vi "Reuben_Reactor_main_jarryd.vi"() -> ()   [LabVIEW 2018]
uses:
  Labview files/Waldo Labview Files/Control 1.ctl
  Labview files/Waldo Labview Files/Control 2.ctl
  <vilib>/DAQmx/read.llb/DAQmx Read (Analog 1D DBL NChan 1Samp).vi
  <vilib>/DAQmx/write.llb/DAQmx Write (Digital 1D Bool NChan 1Samp 1Line).vi
  <vilib>/DAQmx/write.llb/DAQmx Write (Analog 1D DBL NChan 1Samp).vi
  <vilib>/DAQmx/create/channels.llb/DAQmx Create Channel (AI-Current-Basic).vi
  <vilib>/DAQmx/create/channels.llb/DAQmx Create Channel (AI-Voltage-Basic).vi
  <vilib>/DAQmx/create/channels.llb/DAQmx Create Channel (DO-Digital Output).vi
  <vilib>/DAQmx/create/channels.llb/DAQmx Create Channel (AO-Current-Basic).vi
  <vilib>/DAQmx/miscellaneous.llb/DAQmx Fill In Error Info.vi
  <vilib>/Utility/file.llb/Write To Spreadsheet File (string).vi
panel:
  in  "Offset":dbl
  out "Run time":dbl
  out "x*y":dbl
  in  "Numeric":dbl format="%#_13g"
  in  "Actual RPM":dbl format="%#_13g"
  in  "Nitrogen rpm":dbl format="%#_13g"
  in  "Glucose rpm":dbl format="%#_13g"
  in  "Heating cycle (s)":dbl=5.0 format="%#_13g"
  out "Air Average":dbl
  out "Sample Time (ms)":u32=1000
  out "Time":string
  out "On/Off":bool
  out "O2 % Average":dbl
  out "CO2 % Average":dbl
  out "Python code error out":errorcluster
  in  "Inlet O2 %":dbl format="%#_13g"
  in  "Biomass (g)":dbl format="%#_13g"
  in  "Inlet CO2 %":dbl format="%#_13g"
  in  "Python code":path
  out "Data Outputs":dbl[](array[numeric]) format="%.4f"
  in  "323 Auto":bool
  in  "323 Direction":bool
  out "CO2 Average":dbl
  in  "120U Manual":bool
  in  "120U On/Off":bool
  out "Dosing average":dbl
  out "Pump":bool
  in  "Integrator array size":dbl
  in  "Auto":bool
  in  "Heating fraction":dbl
  in  "Temperature setpoint":dbl
  in  "File path (dialog if empty)":path
  out "Data Inputs":T1 format="%.8f"
  in  "Feed rpm \n(0.4623 ml/min/rpm)":dbl
  in  "Gas Recycle":dbl
  in  "Dosing rpm\n (0.042 ml/min/rpm)":dbl
  in  "Broth Recycle":dbl
  in  "Air (ml/min)":dbl
  in  "CO2 (ml/min)":dbl
  in  "Tab Control":enum32{"10 min", "1 h", "6 h", "24 h", "100 h"}(tab)
  out "Gas analyser O2 % 10 min":dbl(graph)
  out "pH 10 min":dbl(graph)
  out "CO2 Feed 10 min":dbl(graph)
  out "Gas analyser CO2 % 10 min":dbl(graph)
  out "Air Feed 10 min":dbl(graph)
  out "blank":dbl(graph)
  out "Temperature 10 min":dbl(graph)
  out "Dosing 10 min":dbl(graph)
  out "O2 rate 10 min":dbl(graph)
  out "CO2 rate 10 min":dbl(graph)
  out "Fumaric acid 10 min":dbl(graph)
  out "Ethanol 10 min":dbl(graph)
  out "blank":dbl(graph)
  out "CO2 Feed 1 h":dbl(graph)
  out "Temperature 1 h":dbl(graph)
  out "pH 1 h":dbl(graph)
  out "Gas analyser O2 % 1 h":dbl(graph)
  out "Air Feed 1 h":dbl(graph)
  out "Gas analyser CO2 % 1 h":dbl(graph)
  out "Dosing 1 h":dbl(graph)
  out "O2 rate 1 h":dbl(graph)
  out "Fumaric acid 1 h":dbl(graph)
  out "CO2 rate 1 h":dbl(graph)
  out "Ethanol 1 h":dbl(graph)
  out "blank":dbl(graph)
  out "Air Feed 6 h":dbl(graph)
  out "Gas analyser O2 % 6 h":dbl(graph)
  out "Gas analyser CO2 % 6 h":dbl(graph)
  out "CO2 Feed 6 h":dbl(graph)
  out "pH 6 h":dbl(graph)
  out "Temperature 6 h":dbl(graph)
  out "Dosing 6 h":dbl(graph)
  out "O2 rate 6 h":dbl(graph)
  out "Fumaric acid 6 h":dbl(graph)
  out "CO2 rate 6 h":dbl(graph)
  out "Ethanol 6 h":dbl(graph)
  out "Temperature 24 h":dbl(graph)
  out "pH 24 h":dbl(graph)
  out "CO2 Feed 24 h":dbl(graph)
  out "Air Feed 24 h":dbl(graph)
  out "blank":dbl(graph)
  out "Gas analyser CO2 % 24 h":dbl(graph)
  out "Gas analyser O2 % 24 h":dbl(graph)
  out "Dosing 24hrs":dbl(graph)
  out "CO2 rate 24 h":dbl(graph)
  out "O2 rate 24 h":dbl(graph)
  out "Fumaric acid 24 h":dbl(graph)
  out "Ethanol 24 h":dbl(graph)
  out "Temperature 100 h":dbl(graph)
  out "pH 100 h":dbl(graph)
  out "CO2 Feed 100 h":dbl(graph)
  out "Air Feed 100 h":dbl(graph)
  out "blank":dbl(graph)
  out "Gas analyser CO2 % 100 h":dbl(graph)
  out "Gas analyser O2 % 100 h":dbl(graph)
  out "Dosing 100hrs":dbl(graph)
  out "O2 rate 100 h":dbl(graph)
  out "CO2 rate 100 h":dbl(graph)
  out "Fumaric acid 100 h":dbl(graph)
  out "Ethanol 100 h":dbl(graph)
  out "Air (ml/min)":dbl
  out "O2 %":dbl
  out "CO2 %":dbl
  out "CO2 (ml/min)":dbl
  out "Temperature":dbl
  out "pH":dbl
  in  "Stop":bool
  # "Gas Analyser"
  # "Python Inputs"
  # "Input variables"
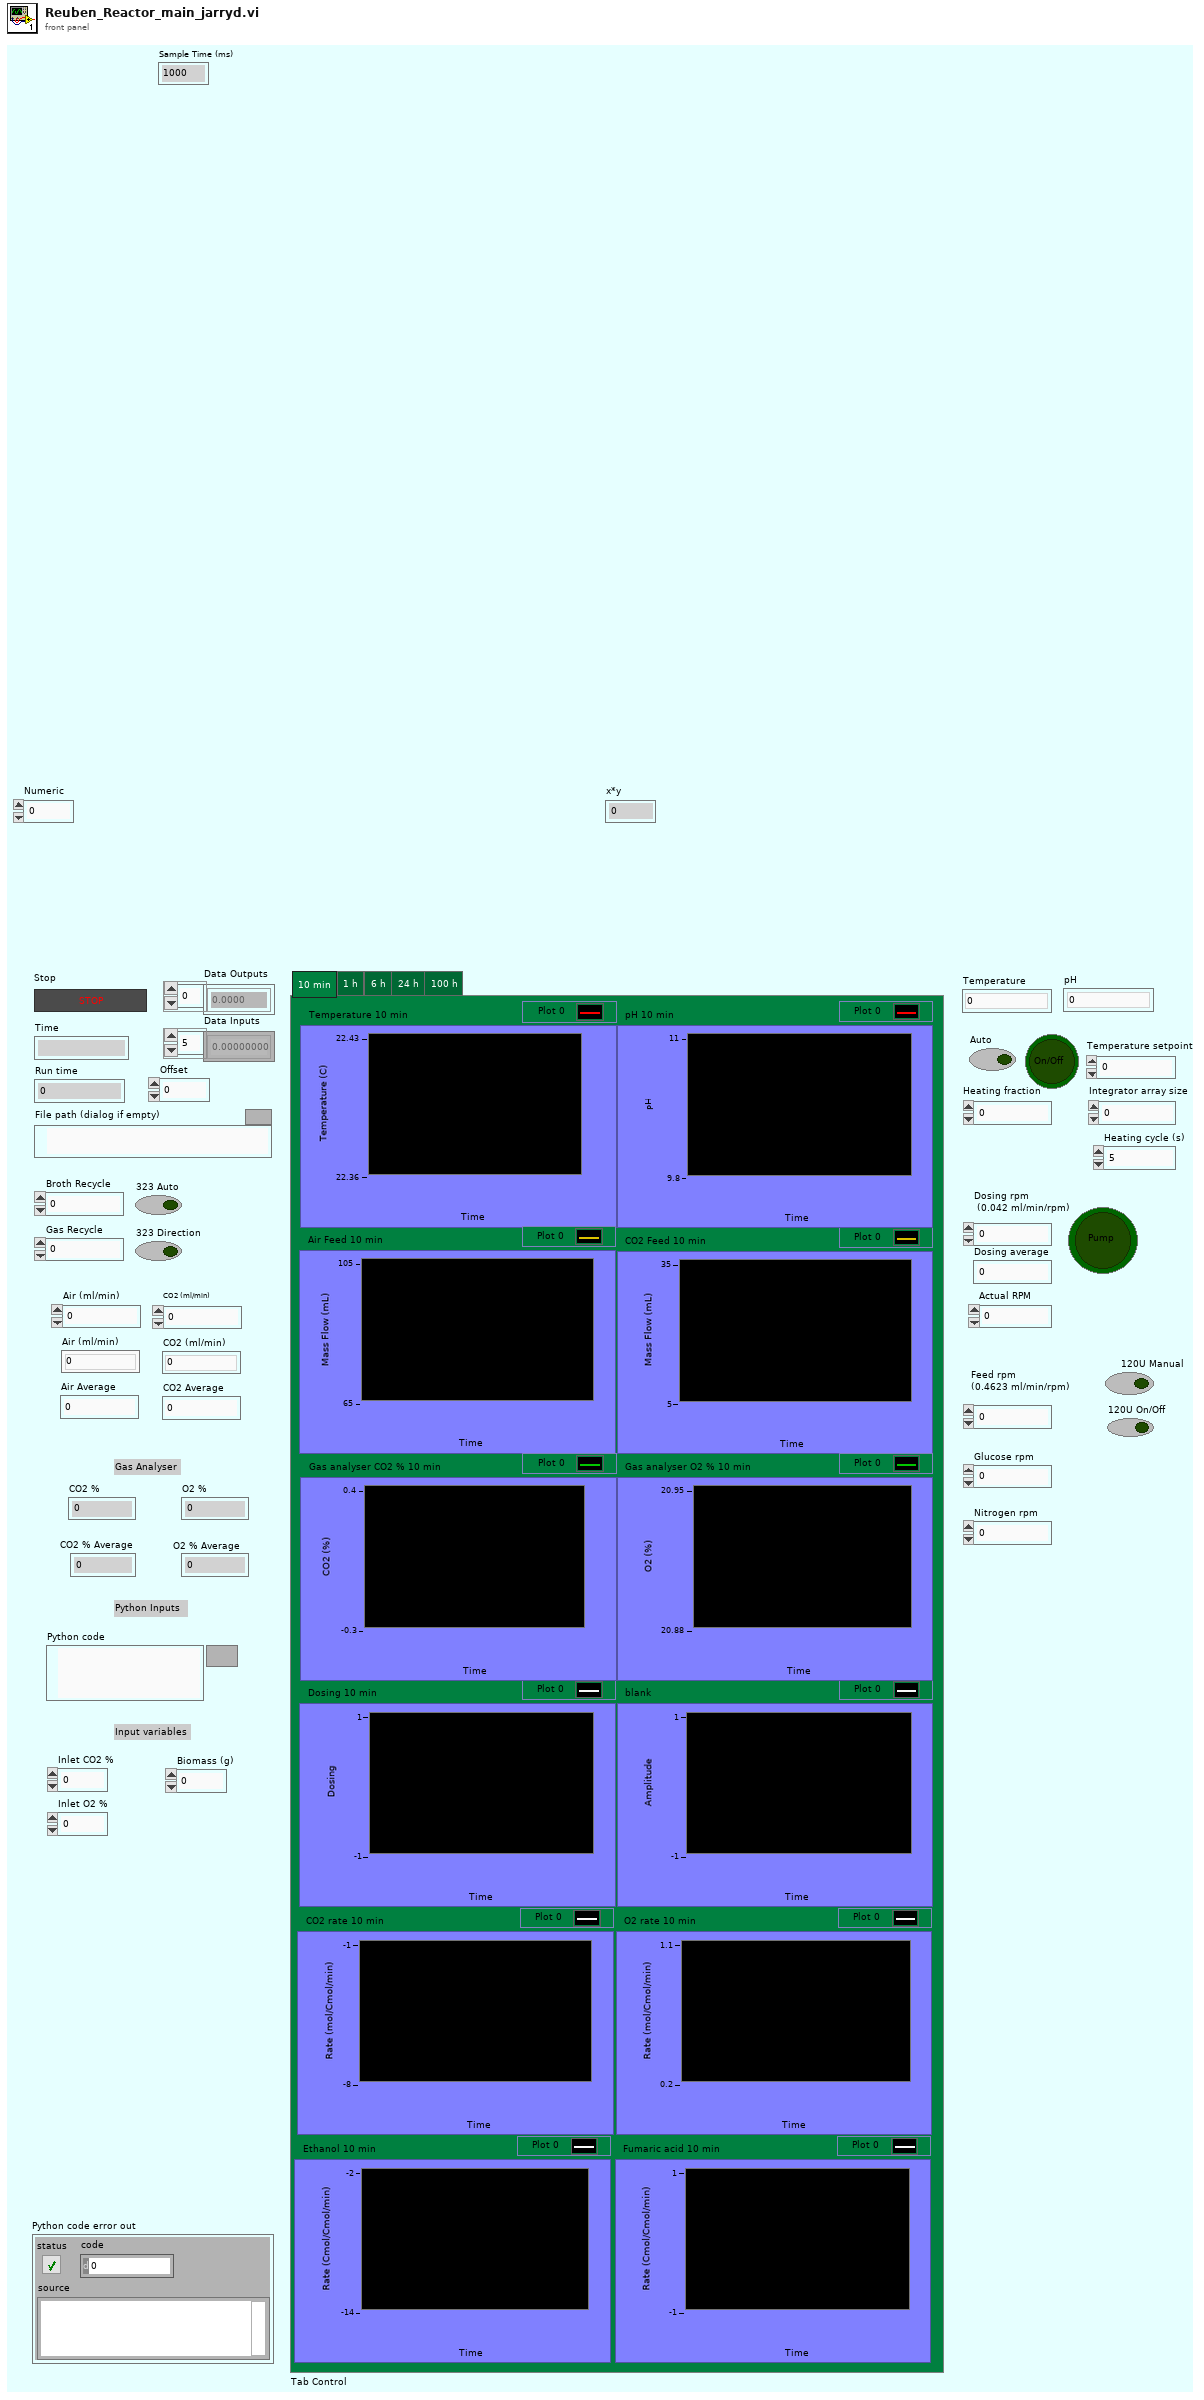
[diagram p1: front panel]
types:
  T1 = typedef "Control 1.ctl" = T2[]
  T2 = typedef "Control 2.ctl" = dbl
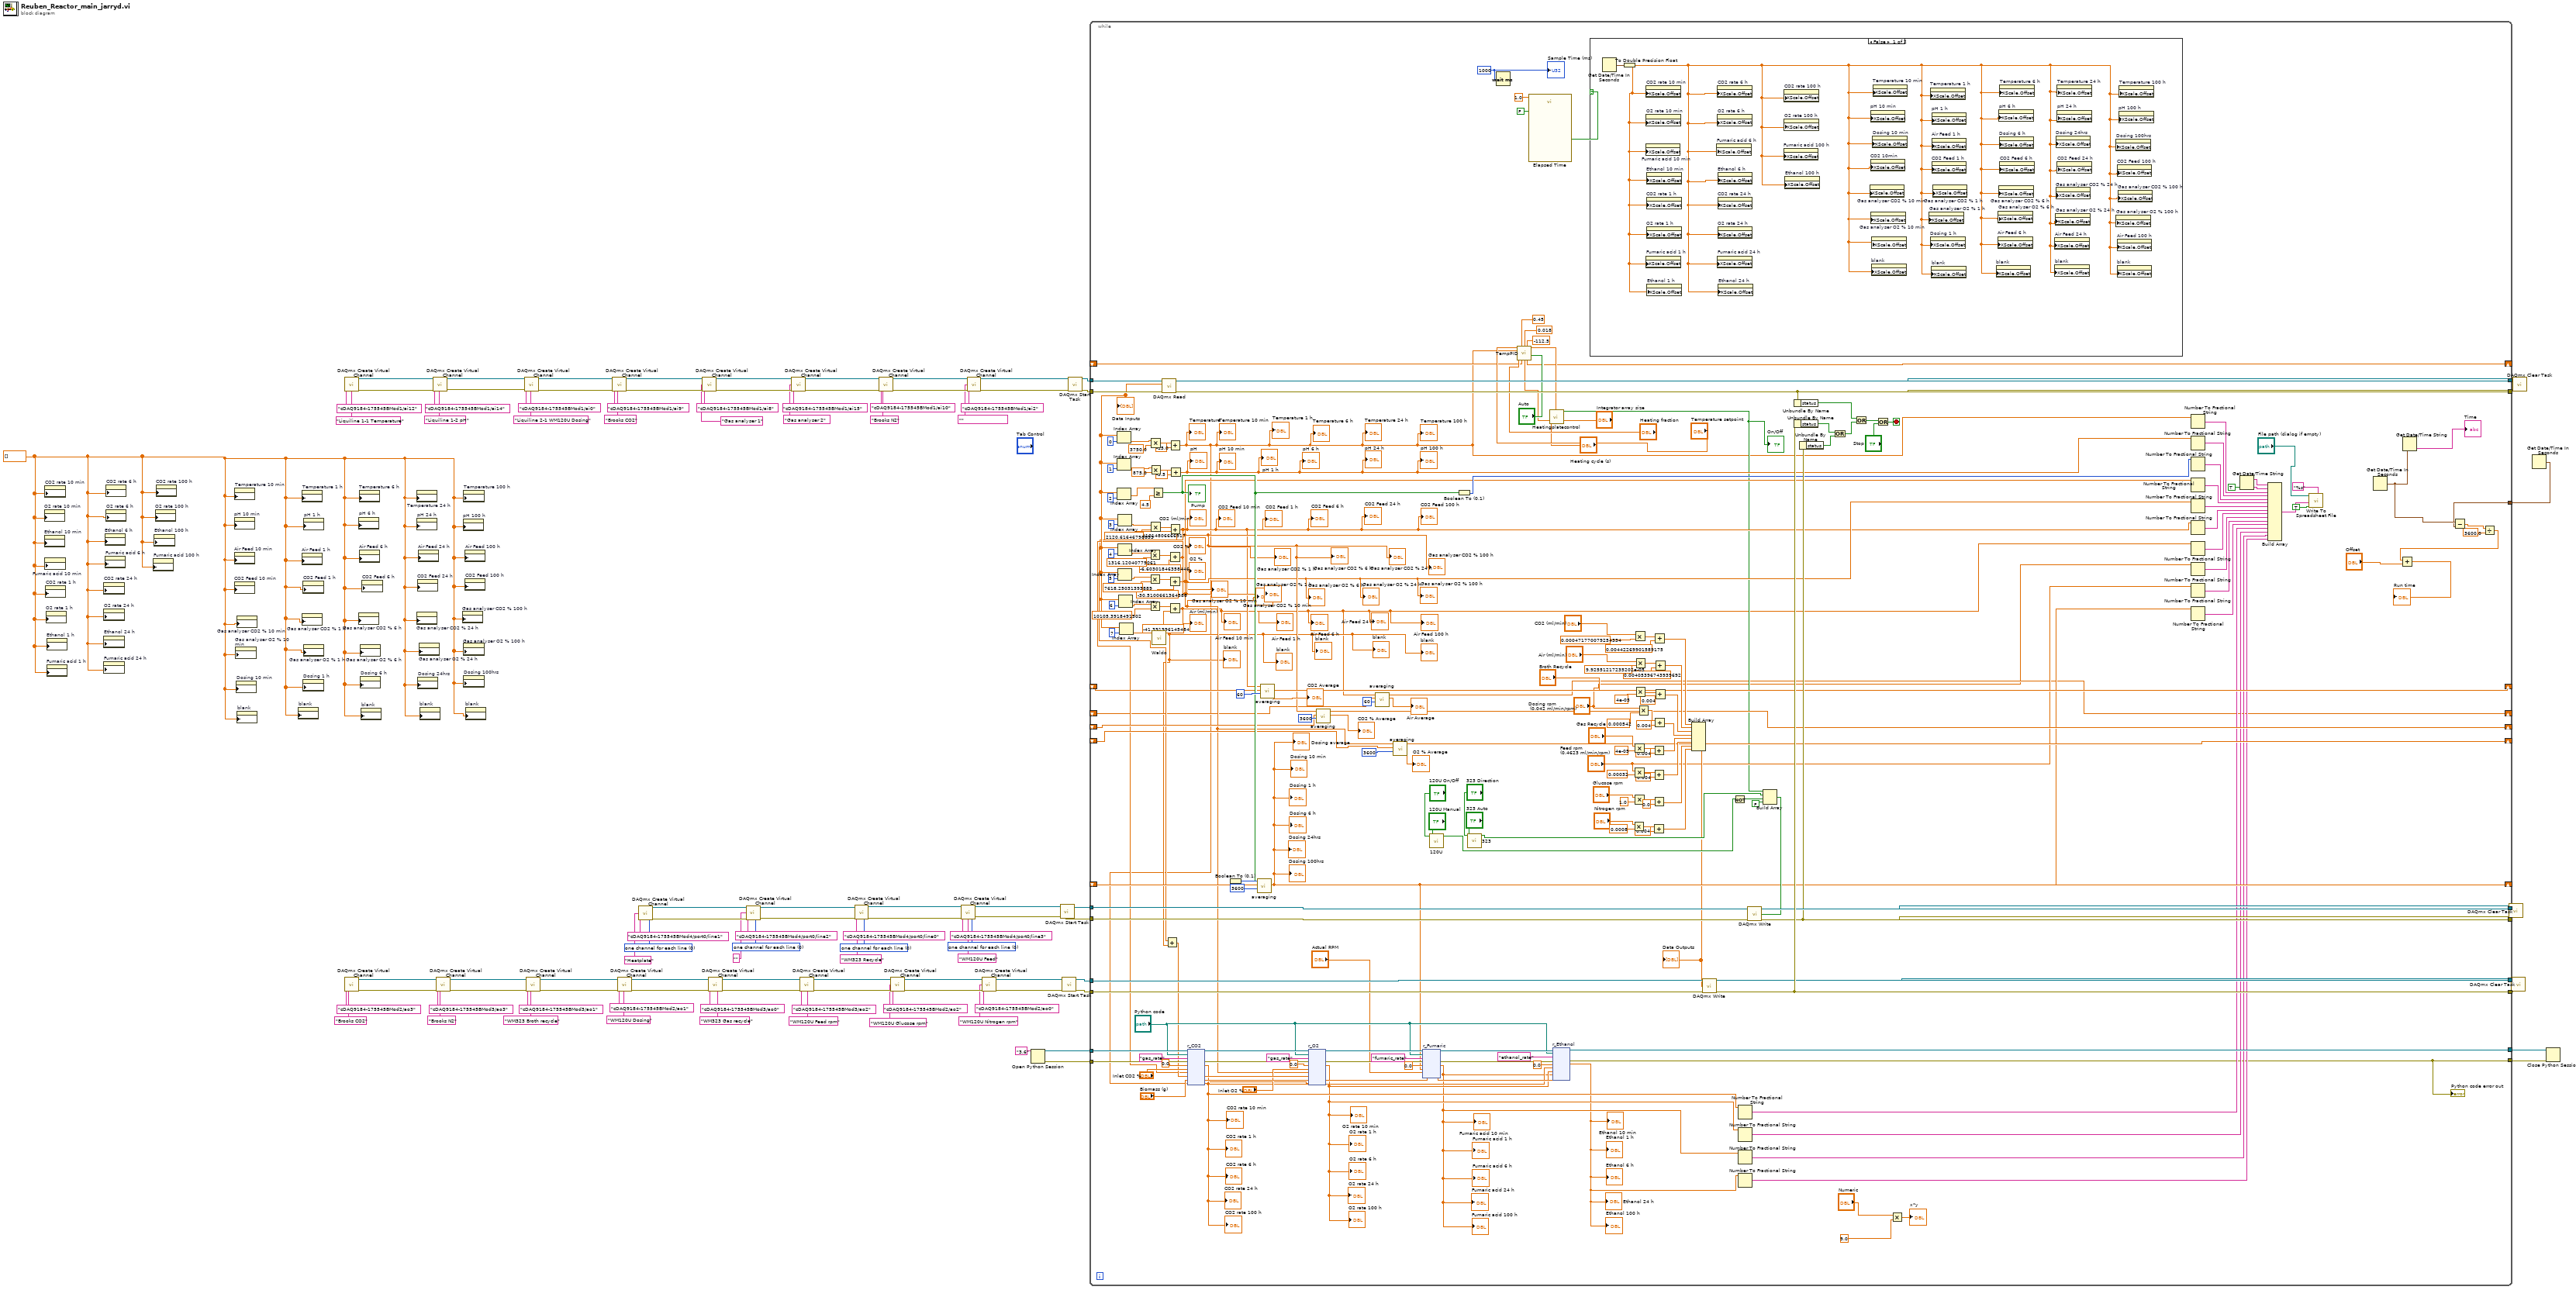
[diagram p0: block diagram]
diagram:
  w2 = dbl[] [] ("History Data")
  w27 = 0 items=["one channel for each line", "one channel for all lines"] ("line grouping")
  w28 = 0 items=["one channel for each line", "one channel for all lines"] ("line grouping")
  w29 = 0 items=["one channel for each line", "one channel for all lines"] ("line grouping")
  w44 = 0 items=["one channel for each line", "one channel for all lines"] ("line grouping")
  n1 = property on="O2 rate 10 min" class="WFChart (strict)"("History Data"=w2) -> ()  [unwired: 2 in, 2 out]
  n2 = property on="Ethanol 10 min" class="WFChart (strict)"("History Data"=w2) -> ()  [unwired: 2 in, 2 out]
  n3 = property on="CO2 rate 10 min" class="WFChart (strict)"("History Data"=w2) -> ()  [unwired: 2 in, 2 out]
  n4 = property on="Fumaric acid 10 min" class="WFChart (strict)"("History Data"=w2) -> ()  [unwired: 2 in, 2 out]
  n5 = property on="CO2 rate 1 h" class="WFChart (strict)"("History Data"=w2) -> ()  [unwired: 2 in, 2 out]
  n6 = property on="O2 rate 1 h" class="WFChart (strict)"("History Data"=w2) -> ()  [unwired: 2 in, 2 out]
  n7 = property on="Ethanol 1 h" class="WFChart (strict)"("History Data"=w2) -> ()  [unwired: 2 in, 2 out]
  n8 = property on="Fumaric acid 1 h" class="WFChart (strict)"("History Data"=w2) -> ()  [unwired: 2 in, 2 out]
  n9 = property on="CO2 rate 24 h" class="WFChart (strict)"("History Data"=w2) -> ()  [unwired: 2 in, 2 out]
  n10 = property on="O2 rate 24 h" class="WFChart (strict)"("History Data"=w2) -> ()  [unwired: 2 in, 2 out]
  n11 = property on="Ethanol 24 h" class="WFChart (strict)"("History Data"=w2) -> ()  [unwired: 2 in, 2 out]
  n12 = property on="Fumaric acid 24 h" class="WFChart (strict)"("History Data"=w2) -> ()  [unwired: 2 in, 2 out]
  n13 = property on="Ethanol 6 h" class="WFChart (strict)"("History Data"=w2) -> ()  [unwired: 2 in, 2 out]
  n14 = property on="Fumaric acid 6 h" class="WFChart (strict)"("History Data"=w2) -> ()  [unwired: 2 in, 2 out]
  n15 = property on="CO2 rate 6 h" class="WFChart (strict)"("History Data"=w2) -> ()  [unwired: 2 in, 2 out]
  n16 = property on="O2 rate 6 h" class="WFChart (strict)"("History Data"=w2) -> ()  [unwired: 2 in, 2 out]
  n17 = property on="Fumaric acid 100 h" class="WFChart (strict)"("History Data"=w2) -> ()  [unwired: 2 in, 2 out]
  n18 = property on="Ethanol 100 h" class="WFChart (strict)"("History Data"=w2) -> ()  [unwired: 2 in, 2 out]
  n19 = property on="O2 rate 100 h" class="WFChart (strict)"("History Data"=w2) -> ()  [unwired: 2 in, 2 out]
  n20 = property on="CO2 rate 100 h" class="WFChart (strict)"("History Data"=w2) -> ()  [unwired: 2 in, 2 out]
  n21 = property on="pH 10 min" class="WFChart (strict)"("History Data"=w2) -> ()  [unwired: 2 in, 2 out]
  n22 = property on="Air Feed 10 min" class="WFChart (strict)"("History Data"=w2) -> ()  [unwired: 2 in, 2 out]
  n23 = property on="CO2 Feed 10 min" class="WFChart (strict)"("History Data"=w2) -> ()  [unwired: 2 in, 2 out]
  n24 = property on="Temperature 10 min" class="WFChart (strict)"("History Data"=w2) -> ()  [unwired: 2 in, 2 out]
  n25 = property on="Gas analyser O2 % 10 min" class="WFChart (strict)"("History Data"=w2) -> ()  [unwired: 2 in, 2 out]
  n26 = property on="Dosing 10 min" class="WFChart (strict)"("History Data"=w2) -> ()  [unwired: 2 in, 2 out]
  n27 = property on="Gas analyser CO2 % 10 min" class="WFChart (strict)"("History Data"=w2) -> ()  [unwired: 2 in, 2 out]
  n28 = property on="blank" class="WFChart (strict)"("History Data"=w2) -> ()  [unwired: 2 in, 2 out]
  n29 = property on="blank" class="WFChart (strict)"("History Data"=w2) -> ()  [unwired: 2 in, 2 out]
  n30 = property on="Air Feed 1 h" class="WFChart (strict)"("History Data"=w2) -> ()  [unwired: 2 in, 2 out]
  n31 = property on="Temperature 1 h" class="WFChart (strict)"("History Data"=w2) -> ()  [unwired: 2 in, 2 out]
  n32 = property on="Gas analyser CO2 % 1 h" class="WFChart (strict)"("History Data"=w2) -> ()  [unwired: 2 in, 2 out]
  n33 = property on="CO2 Feed 1 h" class="WFChart (strict)"("History Data"=w2) -> ()  [unwired: 2 in, 2 out]
  n34 = property on="Dosing 1 h" class="WFChart (strict)"("History Data"=w2) -> ()  [unwired: 2 in, 2 out]
  n35 = property on="pH 1 h" class="WFChart (strict)"("History Data"=w2) -> ()  [unwired: 2 in, 2 out]
  n36 = property on="Gas analyser O2 % 1 h" class="WFChart (strict)"("History Data"=w2) -> ()  [unwired: 2 in, 2 out]
  n37 = call-poly <vilib>:"DAQmx Create Virtual Channel.vi"("physical channels"=tag "cDAQ9184-175545BMod1/ai12", "name to assign"="Liquiline 1-1 Temperature") -> ("task out"=w101:refnum<k21>, "error out"=w100:errorcluster)  [unwired: 12 in]
  n38 = call-poly <vilib>:"DAQmx Create Virtual Channel.vi"("physical channels"=tag "cDAQ9184-175545BMod2/ao3", "name to assign"="Brooks CO2") -> ("task out"=w87:refnum<k21>, "error out"=w86:errorcluster)  [unwired: 12 in]
  n39 = property on="Gas analyser CO2 % 6 h" class="WFChart (strict)"("History Data"=w2) -> ()  [unwired: 2 in, 2 out]
  n40 = property on="pH 6 h" class="WFChart (strict)"("History Data"=w2) -> ()  [unwired: 2 in, 2 out]
  n41 = property on="Temperature 6 h" class="WFChart (strict)"("History Data"=w2) -> ()  [unwired: 2 in, 2 out]
  n42 = property on="Air Feed 6 h" class="WFChart (strict)"("History Data"=w2) -> ()  [unwired: 2 in, 2 out]
  n43 = property on="Gas analyser O2 % 6 h" class="WFChart (strict)"("History Data"=w2) -> ()  [unwired: 2 in, 2 out]
  n44 = property on="Dosing 6 h" class="WFChart (strict)"("History Data"=w2) -> ()  [unwired: 2 in, 2 out]
  n45 = property on="blank" class="WFChart (strict)"("History Data"=w2) -> ()  [unwired: 2 in, 2 out]
  n46 = property on="CO2 Feed 6 h" class="WFChart (strict)"("History Data"=w2) -> ()  [unwired: 2 in, 2 out]
  n47 = property on="Temperature 24 h" class="WFChart (strict)"("History Data"=w2) -> ()  [unwired: 2 in, 2 out]
  n48 = property on="pH 24 h" class="WFChart (strict)"("History Data"=w2) -> ()  [unwired: 2 in, 2 out]
  n49 = property on="Gas analyser CO2 % 24 h" class="WFChart (strict)"("History Data"=w2) -> ()  [unwired: 2 in, 2 out]
  n50 = property on="CO2 Feed 24 h" class="WFChart (strict)"("History Data"=w2) -> ()  [unwired: 2 in, 2 out]
  n51 = property on="Dosing 24hrs" class="WFChart (strict)"("History Data"=w2) -> ()  [unwired: 2 in, 2 out]
  n52 = property on="Air Feed 24 h" class="WFChart (strict)"("History Data"=w2) -> ()  [unwired: 2 in, 2 out]
  n53 = property on="Gas analyser O2 % 24 h" class="WFChart (strict)"("History Data"=w2) -> ()  [unwired: 2 in, 2 out]
  n54 = property on="blank" class="WFChart (strict)"("History Data"=w2) -> ()  [unwired: 2 in, 2 out]
  n55 = call-poly <vilib>:"DAQmx Create Virtual Channel.vi"("task in"=w101, "physical channels"=tag "cDAQ9184-175545BMod1/ai14", "name to assign"="Liquiline 1-2 pH", "error in"=w100) -> ("task out"=w99:refnum<k21>, "error out"=w98:errorcluster)  [unwired: 10 in]
  n56 = call-poly <vilib>:"DAQmx Create Virtual Channel.vi"("task in"=w87, "physical channels"=tag "cDAQ9184-175545BMod3/ao3", "name to assign"="Brooks N2", "error in"=w86) -> ("task out"=w85:refnum<k21>, "error out"=w84:errorcluster)  [unwired: 10 in]
  n57 = property on="Gas analyser CO2 % 100 h" class="WFChart (strict)"("History Data"=w2) -> ()  [unwired: 2 in, 2 out]
  n58 = property on="pH 100 h" class="WFChart (strict)"("History Data"=w2) -> ()  [unwired: 2 in, 2 out]
  n59 = property on="Temperature 100 h" class="WFChart (strict)"("History Data"=w2) -> ()  [unwired: 2 in, 2 out]
  n60 = property on="Gas analyser O2 % 100 h" class="WFChart (strict)"("History Data"=w2) -> ()  [unwired: 2 in, 2 out]
  n61 = property on="Dosing 100hrs" class="WFChart (strict)"("History Data"=w2) -> ()  [unwired: 2 in, 2 out]
  n62 = property on="Air Feed 100 h" class="WFChart (strict)"("History Data"=w2) -> ()  [unwired: 2 in, 2 out]
  n63 = property on="CO2 Feed 100 h" class="WFChart (strict)"("History Data"=w2) -> ()  [unwired: 2 in, 2 out]
  n64 = property on="blank" class="WFChart (strict)"("History Data"=w2) -> ()  [unwired: 2 in, 2 out]
  n65 = call-poly <vilib>:"DAQmx Create Virtual Channel.vi"("task in"=w99, "physical channels"=tag "cDAQ9184-175545BMod1/ai0", "name to assign"="Liquiline 2-1 WM120U Dosing", "error in"=w98) -> ("task out"=w97:refnum<k21>, "error out"=w96:errorcluster)  [unwired: 10 in]
  n66 = call-poly <vilib>:"DAQmx Create Virtual Channel.vi"("task in"=w85, "physical channels"=tag "cDAQ9184-175545BMod3/ao1", "name to assign"="WM323 Broth recycle", "error in"=w84) -> ("task out"=w83:refnum<k21>, "error out"=w82:errorcluster)  [unwired: 10 in]
  n67 = call-poly <vilib>:"DAQmx Create Virtual Channel.vi"("task in"=w97, "physical channels"=tag "cDAQ9184-175545BMod1/ai9", "name to assign"="Brooks CO2", "error in"=w96) -> ("task out"=w95:refnum<k21>, "error out"=w94:errorcluster)  [unwired: 10 in]
  n68 = call-poly <vilib>:"DAQmx Create Virtual Channel.vi"("task in"=w83, "physical channels"=tag "cDAQ9184-175545BMod2/ao1", "name to assign"="WM120U Dosing", "error in"=w82) -> ("task out"=w81:refnum<k21>, "error out"=w80:errorcluster)  [unwired: 10 in]
  n69 = call-poly <vilib>:"DAQmx Create Virtual Channel.vi"("lines"=tag "cDAQ9184-175545BMod4/port0/line1", "name to assign"="Heatplate", "line grouping"=w29) -> ("task out"=w38:refnum<k21>, "error out"=w35:errorcluster)  [unwired: 11 in]
  n70 = call-poly <vilib>:"DAQmx Create Virtual Channel.vi"("task in"=w95, "physical channels"=tag "cDAQ9184-175545BMod1/ai8", "name to assign"="Gas analyser 1", "error in"=w94) -> ("task out"=w93:refnum<k21>, "error out"=w92:errorcluster)  [unwired: 10 in]
  n71 = call-poly <vilib>:"DAQmx Create Virtual Channel.vi"("task in"=w81, "physical channels"=tag "cDAQ9184-175545BMod3/ao0", "name to assign"="WM323 Gas recycle", "error in"=w80) -> ("task out"=w79:refnum<k21>, "error out"=w78:errorcluster)  [unwired: 10 in]
  n72 = call-poly <vilib>:"DAQmx Create Virtual Channel.vi"("task in"=w38, "lines"=tag "cDAQ9184-175545BMod4/port0/line2", "name to assign"="", "line grouping"=w28, "error in"=w35) -> ("task out"=w37:refnum<k21>, "error out"=w34:errorcluster)  [unwired: 9 in]
  n73 = call-poly <vilib>:"DAQmx Create Virtual Channel.vi"("task in"=w93, "physical channels"=tag "cDAQ9184-175545BMod1/ai15", "name to assign"="Gas analyser 2", "error in"=w92) -> ("task out"=w91:refnum<k21>, "error out"=w90:errorcluster)  [unwired: 10 in]
  n74 = call-poly <vilib>:"DAQmx Create Virtual Channel.vi"("task in"=w79, "physical channels"=tag "cDAQ9184-175545BMod3/ao2", "name to assign"="WM120U Feed rpm", "error in"=w78) -> ("task out"=w77:refnum<k21>, "error out"=w76:errorcluster)  [unwired: 10 in]
  n75 = call-poly <vilib>:"DAQmx Create Virtual Channel.vi"("task in"=w37, "lines"=tag "cDAQ9184-175545BMod4/port0/line0", "name to assign"="WM323 Recycle", "line grouping"=w27, "error in"=w34) -> ("task out"=w36:refnum<k21>, "error out"=w33:errorcluster)  [unwired: 9 in]
  n76 = call-poly <vilib>:"DAQmx Create Virtual Channel.vi"("task in"=w91, "physical channels"=tag "cDAQ9184-175545BMod1/ai10", "name to assign"="Brooks N2", "error in"=w90) -> ("task out"=w89:refnum<k21>, "error out"=w88:errorcluster)  [unwired: 10 in]
  n77 = call-poly <vilib>:"DAQmx Create Virtual Channel.vi"("task in"=w77, "physical channels"=tag "cDAQ9184-175545BMod2/ao2", "name to assign"="WM120U Glucose rpm", "error in"=w76) -> ("task out"=w75:refnum<k21>, "error out"=w74:errorcluster)  [unwired: 10 in]
  n78 = call-poly <vilib>:"DAQmx Create Virtual Channel.vi"("task in"=w36, "lines"=tag "cDAQ9184-175545BMod4/port0/line3", "name to assign"="WM120U Feed", "line grouping"=w44, "error in"=w33) -> ("task out"=w43:refnum<k21>, "error out"=w42:errorcluster)  [unwired: 9 in]
  n79 = call-poly <vilib>:"DAQmx Create Virtual Channel.vi"("task in"=w89, "physical channels"=tag "cDAQ9184-175545BMod1/ai2", "name to assign"="", "error in"=w88) -> ("task out"=w73:refnum<k21>, "error out"=w72:errorcluster)  [unwired: 10 in]
  n80 = call-poly <vilib>:"DAQmx Create Virtual Channel.vi"("task in"=w75, "physical channels"=tag "cDAQ9184-175545BMod2/ao0", "name to assign"="WM120U Nitrogen rpm", "error in"=w74) -> ("task out"=w71:refnum<k21>, "error out"=w70:errorcluster)  [unwired: 10 in]
  n81 = Open Python Session(python version="3.6" ("Python version")) -> (session out=w6:refnum<k35>, error out=w7:errorcluster)  [unwired: 2 in]
  n82 = call <vilib>:"DAQmx Start Task.vi"("task/channels in"=w43, "error in"=w42) -> ("task out"=w41:refnum<k21>, "error out"=w40:errorcluster)  [unwired: 12 in]
  n83 = call <vilib>:"DAQmx Start Task.vi"("task/channels in"=w71, "error in"=w70) -> ("task out"=w69:refnum<k21>, "error out"=w68:errorcluster)  [unwired: 12 in]
  n84 = call <vilib>:"DAQmx Start Task.vi"("task/channels in"=w73, "error in"=w72) -> ("task out"=w67:refnum<k21>, "error out"=w66:errorcluster)  [unwired: 12 in]
  n85 = Get Date/Time In Seconds() -> (seconds since 1Jan1904=w1:timestamp)
  n86 = while {
    tunnel: w69 -> [w312]
    tunnel: w68 -> [w311]
    tunnel: w67 -> [w302]
    tunnel: [w314] -> w65
    tunnel: w66 -> [w315]
    tunnel: [w240] -> w63
    tunnel: [w241] -> w62
    tunnel: [w313] -> w64
    tunnel: w41 -> [w219]
    tunnel: w40 -> [w238]
    tunnel: [w237] -> w8
    tunnel: [w229] -> w39
    shift-right: [w220] -> _
    shift-left: _ -> [w225]
    shift-right: [w214] -> _
    shift-left: _ -> [w215]
    shift-right: [w174] -> _
    shift-left: _ -> [w171]
    tunnel: w7 -> [w199]
    tunnel: w6 -> [w195]
    tunnel: [w191] -> w5
    tunnel: [w124] -> w4
    shift-right: [w172] -> _
    shift-left: _ -> [w168]
    shift-right: [w167] -> _
    shift-left: _ -> [w166]
    shift-right: [w123] -> _
    shift-left: _ -> [w122]
    tunnel: w1 -> [w109]
    stop <- w224 stop-if-true
    w161 = u32 1000 ("milliseconds to wait")
    n87 = call-poly <vilib>:"DAQmx Read.vi"("task/channels in"=w302, "error in"=w315) -> ("task out"=w314:refnum<k21>, "data"=w200:dbl[], "error out"=w313:errorcluster)  [unwired: 11 in]
    "Data Inputs" <- w200
    n88 = Index Array(array=w200, index=0) -> (element=w239:dbl)
    n89 = Index Array(array=w200, index=1) -> (element=w283:dbl)
    n90 = Index Array(array=w200, index=2) -> (element=w218:dbl)
    n91 = Index Array(array=w200, index=3) -> (element=w282:dbl)
    n92 = Index Array(array=w200, index=4) -> (element=w281:dbl)
    n93 = Index Array(array=w200, index=5) -> (element=w280:dbl)
    n94 = Index Array(array=w200, index=6) -> (element=w279:dbl)
    n95 = Index Array(array=w200, index=7) -> (element=w278:dbl)
    n96 = Multiply(x=w281, y=1316.12040779061) -> (x*y=w291:dbl)
    n97 = Multiply(x=w280, y=7618.25031393889) -> (x*y=w288:dbl)
    n98 = Multiply(x=w279, y=10105.3918491502) -> (x*y=w285:dbl)
    n99 = Multiply(x=w239, y=3750.0) -> (x*y=w300:dbl)
    n100 = Multiply(x=w282, y=2120.61646798853) -> (x*y=w294:dbl)
    n101 = Multiply(x=w283, y=875.0) -> (x*y=w297:dbl)
    n102 = Greater Or Equal?(x=w218, y=4.5) -> (x >= y?=w205:bool)
    "Pump" <- w205
    n103 = call "Waldo.vi"("Waveform"=w278) -> ("Numeric"=w121:dbl)  [unwired: 10 in]
    "blank" <- w121
    "blank" <- w121
    "blank" <- w121
    "blank" <- w121
    "blank" <- w121
    n104 = Add(x=w291, y=-6.60301846358446) -> (x+y=w141:dbl)
    "CO2 %" <- w141
    "Gas analyser CO2 % 10 min" <- w141
    "Gas analyser CO2 % 6 h" <- w141
    "Gas analyser CO2 % 24 h" <- w141
    "Gas analyser CO2 % 100 h" <- w141
    "Gas analyser CO2 % 1 h" <- w141
    n105 = Add(x=w288, y=-30.5100661364588) -> (x+y=w140:dbl)
    "O2 %" <- w140
    "Gas analyser O2 % 10 min" <- w140
    "Gas analyser O2 % 6 h" <- w140
    "Gas analyser O2 % 24 h" <- w140
    "Gas analyser O2 % 100 h" <- w140
    "Gas analyser O2 % 1 h" <- w140
    n106 = Add(x=w285, y=-41.3919961454843) -> (x+y=w118:dbl)
    "Air (ml/min)" <- w118
    "Air Feed 10 min" <- w118
    "Air Feed 6 h" <- w118
    "Air Feed 24 h" <- w118
    "Air Feed 100 h" <- w118
    "Air Feed 1 h" <- w118
    n107 = Add(x=w300, y=-15.0) -> (x+y=w117:dbl)
    "Temperature" <- w117
    "Temperature 6 h" <- w117
    "Temperature 24 h" <- w117
    "Temperature 100 h" <- w117
    "Temperature 10 min" <- w117
    "Temperature 1 h" <- w117
    n108 = Add(x=w294, y=-9.41014806666917) -> (x+y=w139:dbl)
    "CO2 (ml/min)" <- w139
    "CO2 Feed 10 min" <- w139
    "CO2 Feed 6 h" <- w139
    "CO2 Feed 24 h" <- w139
    "CO2 Feed 100 h" <- w139
    "CO2 Feed 1 h" <- w139
    n109 = Add(x=w139, y=w121) -> (x+y=w180:dbl)
    n110 = Add(x=w297, y=-3.5) -> (x+y=w135:dbl)
    "pH" <- w135
    "pH 10 min" <- w135
    "pH 6 h" <- w135
    "pH 24 h" <- w135
    "pH 100 h" <- w135
    "pH 1 h" <- w135
    n111 = node "r_CO2"(w195, "Python code", "gas_rate" ("function name"), w199, 0.0, "Inlet CO2 %", w141, w180, "Biomass (g)", w117) -> (w194:refnum<k35>, w198:errorcluster, w133:dbl, w178:dbl, w116:dbl)  [unwired: 3 in, 2 out]
    "CO2 rate 10 min" <- w133
    "CO2 rate 6 h" <- w133
    "CO2 rate 24 h" <- w133
    "CO2 rate 100 h" <- w133
    "CO2 rate 1 h" <- w133
    n112 = Boolean To (0,1)(Boolean=w205) -> (0, 1=w216:i16)
    n113 = call "averaging.vi"("Averaging Time"=3600, "Array in"=w215, "Input"=w216) -> ("Average"=w137:dbl, "Array out"=w214:dbl[])  [unwired: 7 in]
    "Dosing average" <- w137
    "Dosing 10 min" <- w137
    "Dosing 6 h" <- w137
    "Dosing 24hrs" <- w137
    "Dosing 100hrs" <- w137
    "Dosing 1 h" <- w137
    n114 = call "averaging.vi"("Averaging Time"=60, "Array in"=w171, "Input"=w139) -> ("Average"=→"CO2 Average":dbl, "Array out"=w174:dbl[])  [unwired: 7 in]
    n115 = node "r_O2"(w194, "Python code", "gas_rate" ("function name"), w198, 0.0, "Inlet O2 %", w140, w180, w178, w116) -> (w193:refnum<k35>, w197:errorcluster, w132:dbl, w177:dbl)  [unwired: 4 in, 2 out]
    "O2 rate 10 min" <- w132
    "O2 rate 6 h" <- w132
    "O2 rate 24 h" <- w132
    "O2 rate 100 h" <- w132
    "O2 rate 1 h" <- w132
    n116 = call "averaging.vi"("Averaging Time"=3600, "Array in"=w168, "Input"=w141) -> ("Average"=→"CO2 % Average":dbl, "Array out"=w172:dbl[])  [unwired: 7 in]
    n117 = call "averaging.vi"("Averaging Time"=60, "Array in"=w122, "Input"=w118) -> ("Average"=→"Air Average":dbl, "Array out"=w123:dbl[])  [unwired: 7 in]
    n118 = call "averaging.vi"("Averaging Time"=3600, "Array in"=w166, "Input"=w140) -> ("Average"=→"O2 % Average":dbl, "Array out"=w167:dbl[])  [unwired: 7 in]
    n119 = node "r_Fumaric"(w193, "Python code", "fumaric_rate" ("function name"), w197, 0.0, w137, "Actual RPM", w177) -> (w192:refnum<k35>, w196:errorcluster, w131:dbl, w176:dbl)  [unwired: 2 in, 2 out]
    "Fumaric acid 10 min" <- w131
    "Fumaric acid 6 h" <- w131
    "Fumaric acid 24 h" <- w131
    "Fumaric acid 100 h" <- w131
    "Fumaric acid 1 h" <- w131
    n120 = call "120U.vi"("Auto"="120U Manual", "Pump On/Off in"="120U On/Off") -> ("Pump On/Off out"=w202:bool)  [unwired: 9 in]
    n121 = Boolean To (0,1)(Boolean=w205) -> (0, 1=w142:i16)
    n122 = call "323.vi"("Auto"="323 Auto", "Pump On/Off in"="323 Direction") -> ("Pump On/Off out"=w206:bool)  [unwired: 9 in]
    n123 = Wait (ms)(milliseconds to wait=w161) -> ()  [unwired: 1 out]
    n124 = call "TempPID.vi"("Temperature setpoint"="Temperature setpoint", "Kp"=0.45, "Ki"=0.018, "Kd"=-112.5, "Temperature in"=w117, "Manual heating fraction"="Heating fraction", "Auto"="Auto", "Array in"=w225, "Integrator array size"="Integrator array size") -> ("Heating fraction"=w232:dbl, "Array out"=w220:dbl[])  [unwired: 4 in, 1 out]
    n125 = call "Elapsed Time"("Time Target (s)"=1.0, "Auto Reset"=FALSE) -> ("Time has Elapsed"=w158:bool)  [unwired: 10 in, 7 out]
    n126 = call "Heatingplatecontrol.vi"("Heating cycle (s)"="Heating cycle (s)", "Heating fraction"=w232) -> ("Heating plate on"=w125:bool)  [unwired: 9 in]
    "On/Off" <- w125
    n127 = node "r_Ethanol"(w192, "Python code", "ethanol_rate" ("function name"), w196, 0.0, w133, w132, w131, w176) -> (w191:refnum<k35>, w124:errorcluster, w130:dbl)  [unwired: 4 in, 2 out]
    "Ethanol 10 min" <- w130
    "Ethanol 6 h" <- w130
    "Ethanol 24 h" <- w130
    "Ethanol 100 h" <- w130
    "Ethanol 1 h" <- w130
    "Python code error out" <- w124
    n128 = case shown="False" w158 {
      frame False {
        n129 = Get Date/Time In Seconds() -> (seconds since 1Jan1904=w320:timestamp)
        n130 = To Double Precision Float(number=w320) -> (double precision float=w319:dbl)
        n131 = property on="Fumaric acid 10 min" class="WFChart (strict)"("XScale.Offset"=w319) -> ()  [unwired: 2 in, 2 out]
        n132 = property on="CO2 rate 10 min" class="WFChart (strict)"("XScale.Offset"=w319) -> ()  [unwired: 2 in, 2 out]
        n133 = property on="O2 rate 10 min" class="WFChart (strict)"("XScale.Offset"=w319) -> ()  [unwired: 2 in, 2 out]
        n134 = property on="Fumaric acid 1 h" class="WFChart (strict)"("XScale.Offset"=w319) -> ()  [unwired: 2 in, 2 out]
        n135 = property on="Ethanol 10 min" class="WFChart (strict)"("XScale.Offset"=w319) -> ()  [unwired: 2 in, 2 out]
        n136 = property on="CO2 rate 1 h" class="WFChart (strict)"("XScale.Offset"=w319) -> ()  [unwired: 2 in, 2 out]
        n137 = property on="O2 rate 1 h" class="WFChart (strict)"("XScale.Offset"=w319) -> ()  [unwired: 2 in, 2 out]
        n138 = property on="Ethanol 1 h" class="WFChart (strict)"("XScale.Offset"=w319) -> ()  [unwired: 2 in, 2 out]
        n139 = property on="Fumaric acid 6 h" class="WFChart (strict)"("XScale.Offset"=w319) -> ()  [unwired: 2 in, 2 out]
        n140 = property on="CO2 rate 6 h" class="WFChart (strict)"("XScale.Offset"=w319) -> ()  [unwired: 2 in, 2 out]
        n141 = property on="O2 rate 6 h" class="WFChart (strict)"("XScale.Offset"=w319) -> ()  [unwired: 2 in, 2 out]
        n142 = property on="Fumaric acid 24 h" class="WFChart (strict)"("XScale.Offset"=w319) -> ()  [unwired: 2 in, 2 out]
        n143 = property on="Ethanol 6 h" class="WFChart (strict)"("XScale.Offset"=w319) -> ()  [unwired: 2 in, 2 out]
        n144 = property on="CO2 rate 24 h" class="WFChart (strict)"("XScale.Offset"=w319) -> ()  [unwired: 2 in, 2 out]
        n145 = property on="O2 rate 24 h" class="WFChart (strict)"("XScale.Offset"=w319) -> ()  [unwired: 2 in, 2 out]
        n146 = property on="Ethanol 24 h" class="WFChart (strict)"("XScale.Offset"=w319) -> ()  [unwired: 2 in, 2 out]
        n147 = property on="Fumaric acid 100 h" class="WFChart (strict)"("XScale.Offset"=w319) -> ()  [unwired: 2 in, 2 out]
        n148 = property on="CO2 rate 100 h" class="WFChart (strict)"("XScale.Offset"=w319) -> ()  [unwired: 2 in, 2 out]
        n149 = property on="O2 rate 100 h" class="WFChart (strict)"("XScale.Offset"=w319) -> ()  [unwired: 2 in, 2 out]
        n150 = property on="Ethanol 100 h" class="WFChart (strict)"("XScale.Offset"=w319) -> ()  [unwired: 2 in, 2 out]
        n151 = property on="Gas analyser CO2 % 10 min" class="WFChart (strict)"("XScale.Offset"=w319) -> ()  [unwired: 2 in, 2 out]
        n152 = property on="pH 10 min" class="WFChart (strict)"("XScale.Offset"=w319) -> ()  [unwired: 2 in, 2 out]
        n153 = property on="CO2 10min" class="WFChart (strict)"("XScale.Offset"=w319) -> ()  [unwired: 2 in, 2 out]
        n154 = property on="Gas analyser O2 % 10 min" class="WFChart (strict)"("XScale.Offset"=w319) -> ()  [unwired: 2 in, 2 out]
        n155 = property on="blank" class="WFChart (strict)"("XScale.Offset"=w319) -> ()  [unwired: 2 in, 2 out]
        n156 = property class="WFChart (strict)"("XScale.Offset"=w319) -> ()  [unwired: 2 in, 2 out]
        n157 = property on="Dosing 10 min" class="WFChart (strict)"("XScale.Offset"=w319) -> ()  [unwired: 2 in, 2 out]
        n158 = property on="Temperature 10 min" class="WFChart (strict)"("XScale.Offset"=w319) -> ()  [unwired: 2 in, 2 out]
        n159 = property on="Gas analyser O2 % 1 h" class="WFChart (strict)"("XScale.Offset"=w319) -> ()  [unwired: 2 in, 2 out]
        n160 = property on="Temperature 1 h" class="WFChart (strict)"("XScale.Offset"=w319) -> ()  [unwired: 2 in, 2 out]
        n161 = property on="Dosing 1 h" class="WFChart (strict)"("XScale.Offset"=w319) -> ()  [unwired: 2 in, 2 out]
        n162 = property on="blank" class="WFChart (strict)"("XScale.Offset"=w319) -> ()  [unwired: 2 in, 2 out]
        n163 = property on="pH 1 h" class="WFChart (strict)"("XScale.Offset"=w319) -> ()  [unwired: 2 in, 2 out]
        n164 = property on="Air Feed 1 h" class="WFChart (strict)"("XScale.Offset"=w319) -> ()  [unwired: 2 in, 2 out]
        n165 = property on="CO2 Feed 1 h" class="WFChart (strict)"("XScale.Offset"=w319) -> ()  [unwired: 2 in, 2 out]
        n166 = property on="Gas analyser CO2 % 1 h" class="WFChart (strict)"("XScale.Offset"=w319) -> ()  [unwired: 2 in, 2 out]
        n167 = property on="blank" class="WFChart (strict)"("XScale.Offset"=w319) -> ()  [unwired: 2 in, 2 out]
        n168 = property on="Air Feed 6 h" class="WFChart (strict)"("XScale.Offset"=w319) -> ()  [unwired: 2 in, 2 out]
        n169 = property on="Gas analyser O2 % 6 h" class="WFChart (strict)"("XScale.Offset"=w319) -> ()  [unwired: 2 in, 2 out]
        n170 = property on="pH 6 h" class="WFChart (strict)"("XScale.Offset"=w319) -> ()  [unwired: 2 in, 2 out]
        n171 = property on="Gas analyser CO2 % 6 h" class="WFChart (strict)"("XScale.Offset"=w319) -> ()  [unwired: 2 in, 2 out]
        n172 = property on="Dosing 6 h" class="WFChart (strict)"("XScale.Offset"=w319) -> ()  [unwired: 2 in, 2 out]
        n173 = property on="Temperature 6 h" class="WFChart (strict)"("XScale.Offset"=w319) -> ()  [unwired: 2 in, 2 out]
        n174 = property on="CO2 Feed 6 h" class="WFChart (strict)"("XScale.Offset"=w319) -> ()  [unwired: 2 in, 2 out]
        n175 = property on="Air Feed 24 h" class="WFChart (strict)"("XScale.Offset"=w319) -> ()  [unwired: 2 in, 2 out]
        n176 = property on="blank" class="WFChart (strict)"("XScale.Offset"=w319) -> ()  [unwired: 2 in, 2 out]
        n177 = property on="Gas analyser O2 % 24 h" class="WFChart (strict)"("XScale.Offset"=w319) -> ()  [unwired: 2 in, 2 out]
        n178 = property on="Dosing 24hrs" class="WFChart (strict)"("XScale.Offset"=w319) -> ()  [unwired: 2 in, 2 out]
        n179 = property on="Gas analyser CO2 % 24 h" class="WFChart (strict)"("XScale.Offset"=w319) -> ()  [unwired: 2 in, 2 out]
        n180 = property on="Temperature 24 h" class="WFChart (strict)"("XScale.Offset"=w319) -> ()  [unwired: 2 in, 2 out]
        n181 = property on="pH 24 h" class="WFChart (strict)"("XScale.Offset"=w319) -> ()  [unwired: 2 in, 2 out]
        n182 = property on="CO2 Feed 24 h" class="WFChart (strict)"("XScale.Offset"=w319) -> ()  [unwired: 2 in, 2 out]
        n183 = property on="Dosing 100hrs" class="WFChart (strict)"("XScale.Offset"=w319) -> ()  [unwired: 2 in, 2 out]
        n184 = property on="Gas analyser O2 % 100 h" class="WFChart (strict)"("XScale.Offset"=w319) -> ()  [unwired: 2 in, 2 out]
        n185 = property on="CO2 Feed 100 h" class="WFChart (strict)"("XScale.Offset"=w319) -> ()  [unwired: 2 in, 2 out]
        n186 = property on="Air Feed 100 h" class="WFChart (strict)"("XScale.Offset"=w319) -> ()  [unwired: 2 in, 2 out]
        n187 = property on="blank" class="WFChart (strict)"("XScale.Offset"=w319) -> ()  [unwired: 2 in, 2 out]
        n188 = property on="Gas analyser CO2 % 100 h" class="WFChart (strict)"("XScale.Offset"=w319) -> ()  [unwired: 2 in, 2 out]
        n189 = property on="pH 100 h" class="WFChart (strict)"("XScale.Offset"=w319) -> ()  [unwired: 2 in, 2 out]
        n190 = property on="Temperature 100 h" class="WFChart (strict)"("XScale.Offset"=w319) -> ()  [unwired: 2 in, 2 out]
      }
      frame True {
      }
    }
    n191 = Multiply(x="Nitrogen rpm", y=0.0008) -> (x*y=w255:dbl)
    n192 = Multiply(x="Gas Recycle", y=4e-05) -> (x*y=w264:dbl)
    n193 = Multiply(x="Feed rpm \n(0.4623 ml/min/rpm)", y=0.00032) -> (x*y=w261:dbl)
    n194 = Multiply(x="Glucose rpm", y=1.0) -> (x*y=w258:dbl)
    n195 = Multiply(x="CO2 (ml/min)", y=0.000471770079254334) -> (x*y=w276:dbl)
    n196 = Multiply(x="Air (ml/min)", y=9.92551217235202e-05) -> (x*y=w273:dbl)
    n197 = Multiply(x="Broth Recycle", y=4e-05) -> (x*y=w270:dbl)
    n198 = Multiply(x="Dosing rpm\n (0.042 ml/min/rpm)", y=0.000542) -> (x*y=w267:dbl)
    n199 = Add(x=w255, y=0.004) -> (x+y=w246:dbl)
    n200 = Add(x=w264, y=0.004) -> (x+y=w249:dbl)
    n201 = Add(x=w261, y=0.004) -> (x+y=w248:dbl)
    n202 = Add(x=w258, y=0.0) -> (x+y=w247:dbl)
    n203 = Add(x=w276, y=0.00442269901589175) -> (x+y=w253:dbl)
    n204 = Add(x=w267, y=0.004) -> (x+y=w250:dbl)
    n205 = Add(x=w273, y=0.00405396743939692) -> (x+y=w252:dbl)
    n206 = Add(x=w270, y=0.004) -> (x+y=w251:dbl)
    n207 = Build Array(w253, w252, w251, w250, w249, w248, w247, w246) -> (w201:dbl[])
    "Data Outputs" <- w201
    n208 = call-poly <vilib>:"DAQmx Write.vi"("task/channels in"=w312, "data"=w201, "error in"=w311) -> ("task out"=w240:refnum<k21>, "error out"=w241:errorcluster)  [unwired: 10 in, 1 out]
    n209 = Not(x=w202) -> (.not. x?=w211:bool)
    n210 = Number To Fractional String(number=w133) -> (F-format string=w129:string)  [unwired: 3 in]
    n211 = Number To Fractional String(number=w132) -> (F-format string=w128:string)  [unwired: 3 in]
    n212 = Number To Fractional String(number=w131) -> (F-format string=w127:string)  [unwired: 3 in]
    n213 = Number To Fractional String(number=w130) -> (F-format string=w126:string)  [unwired: 3 in]
    n214 = Build Array(w125, w206, w211, FALSE ("element")) -> (w230:bool[])
    n215 = call-poly <vilib>:"DAQmx Write.vi"("task/channels in"=w219, "data"=w230, "error in"=w238) -> ("task out"=w237:refnum<k21>, "error out"=w229:errorcluster)  [unwired: 10 in, 1 out]
    n216 = Unbundle By Name(w313) -> ("status"=w318:bool)
    n217 = Unbundle By Name(w241) -> ("status"=w227:bool)
    n218 = Unbundle By Name(w229) -> ("status"=w228:bool)
    n219 = Or(x=w227, y=w228) -> (x .or. y?=w226:bool)
    n220 = Or(x=w318, y=w226) -> (x .or. y?=w317:bool)
    n221 = Or(x=w317, y="Stop") -> (x .or. y?=w224:bool)
    n222 = Multiply(x="Numeric", y=9.0) -> (x*y=→"x*y":dbl)
    n223 = Number To Fractional String(number=w117) -> (F-format string=w151:string)  [unwired: 3 in]
    n224 = Number To Fractional String(number=w135) -> (F-format string=w146:string)  [unwired: 3 in]
    n225 = Number To Fractional String(number=w142) -> (F-format string=w150:string)  [unwired: 3 in]
    n226 = Number To Fractional String(number=w141) -> (F-format string=w149:string)  [unwired: 3 in]
    n227 = Number To Fractional String(number=w140) -> (F-format string=w148:string)  [unwired: 3 in]
    n228 = Number To Fractional String(number=w139) -> (F-format string=w147:string)  [unwired: 3 in]
    n229 = Number To Fractional String(number=w118) -> (F-format string=w145:string)  [unwired: 3 in]
    n230 = Number To Fractional String(number="Dosing rpm\n (0.042 ml/min/rpm)") -> (F-format string=w134:string)  [unwired: 3 in]
    n231 = Number To Fractional String(number="Feed rpm \n(0.4623 ml/min/rpm)") -> (F-format string=w144:string)  [unwired: 3 in]
    n232 = Number To Fractional String(number=w137) -> (F-format string=w143:string)  [unwired: 3 in]
    n233 = Get Date/Time String(want seconds? (F)=TRUE) -> (date string=w156:string, time string=w155:string)  [unwired: 2 in]
    n234 = Build Array(w156, w155, w151, w146, w150, w149, w148, w147, w145, w134, w144, w143, w129, w128, w127, w126) -> (w154:string[])
    n235 = call-poly <vilib>:"Write To Spreadsheet File.vi"("format (%s)"="%s", "append to file? (new file:F)"=TRUE, "1D data"=w154, "file path (dialog if empty)"="File path (dialog if empty)") -> ()  [unwired: 4 in, 1 out]
    n236 = Get Date/Time In Seconds() -> (seconds since 1Jan1904=w110:timestamp)
    n237 = Get Date/Time String(seconds (now)=w110) -> (time string=→"Time":string)  [unwired: 2 in, 1 out]
    n238 = Subtract(x=w110, y=w109) -> (x-y=w107:dbl)
    n239 = Divide(x=w107, y=3600.0) -> (x/y=w106:dbl)
    n240 = Add(x=w106, y="Offset") -> (x+y=→"Run time":dbl)
    "Sample Time (ms)" <- w161
  }
  n241 = call <vilib>:"DAQmx Clear Task.vi"("task in"=w8, "error in"=w39) -> ()  [unwired: 13 in, 1 out]
  n242 = call <vilib>:"DAQmx Clear Task.vi"("task in"=w63, "error in"=w62) -> ()  [unwired: 13 in, 1 out]
  n243 = call <vilib>:"DAQmx Clear Task.vi"("task in"=w65, "error in"=w64) -> ()  [unwired: 13 in, 1 out]
  n244 = Close Python Session(session in=w5, error in=w4) -> ()  [unwired: 1 out]
